vi "blokada wysylania manipulatora.vi"(6 "Y":i32, 8 "Zaxis":i32, 9 "X axis":i32, 11 "Boolean in":refnum<vi>) -> (0 "zakres Z":bool, 1 "zakres X":bool, 3 "blokadaa":bool, 4 "zakres Y":bool)   [LabVIEW 2014]
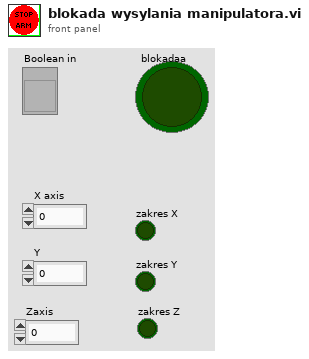
[diagram p1: front panel]
types:
  T1 = enum16{"Rising Edge", "Falling Edge", "Any Edge"}
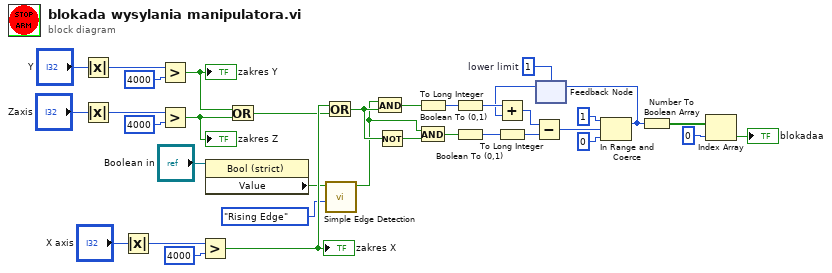
[diagram p0: block diagram]
diagram:
  w1 = 1  # lower limit
  n1 = Absolute Value(x="Y") -> (abs(x)=w31:i32)
  n2 = Absolute Value(x="Zaxis") -> (abs(x)=w11:i32)
  n3 = Absolute Value(x="X axis") -> (abs(x)=w15:i32)
  n4 = Greater?(x=w31, y=4000) -> (0:w8:bool)
  "zakres Y" <- w8
  n5 = Greater?(x=w11, y=4000) -> (0:w10:bool)
  "zakres Z" <- w10
  n6 = Greater?(x=w15, y=4000) -> (0:w32:bool)
  "zakres X" <- w32
  n7 = property class="Bool (strict)"(reference="Boolean in") -> ("Value"=w17:bool)  [unwired: 1 in, 2 out]
  n8 = Or(x=w8, y=w10) -> (x .or. y?=w9:bool)
  n9 = Or(x=w32, y=w9) -> (x .or. y?=w33:bool)
  n10 = call "Simple Edge Detection.vi"("Mode"=T1."Rising Edge", "clk_in"=w17) -> ("edge?"=w24:bool)  [unwired: 9 in]
  n11 = And(x=w24, y=w33) -> (x .and. y?=w19:bool)
  n12 = Not(x=w33) -> (.not. x?=w23:bool)
  n13 = Boolean To (0,1)(Boolean=w19) -> (0, 1=w6:i16)
  n14 = And(x=w24, y=w23) -> (x .and. y?=w22:bool)
  n15 = To Long Integer(number=w6) -> (32bit integer=w7:i32)
  n16 = Boolean To (0,1)(Boolean=w22) -> (0, 1=w4:i16)
  n17 = To Long Integer(number=w4) -> (32bit integer=w5:i32)
  n18 = feedback #1(w1) -> (w3:i32)
  n19 = Add(x=w7, y=w3) -> (x+y=w26:i32)
  n20 = Subtract(x=w26, y=w5) -> (x-y=w25:i32)
  n21 = In Range and Coerce(upper limit=1 ("lower limit"), x=w25, lower limit=0) -> (coerced(x)=w2:i32)  [unwired: 1 out]
  n22 = feedback-in #1(w2) -> ()
  n23 = Number To Boolean Array(number=w2) -> (Boolean array=w27:bool[])
  n24 = Index Array(array=w27, index=0) -> (element=→"blokadaa":bool)
